vi "My Custom Controls - Custom.vi"() -> ()   [LabVIEW 2016]
doc: "Sample numeric display item."
uses:
  <vilib>/NI Veristand/Display Template Support/Display Template Support.llb/cluster_Screen Item Settings.ctl
  <vilib>/NI Veristand/Display Template Support/Display Template Support.llb/cluster_Graph Scale Settings.ctl
  <vilib>/NI Veristand/Display Template Support/Display Template Support.llb/cluster_Graph Plot Settings.ctl
  _typedefs/Custom Control_Data.ctl
  <vilib>/NI Veristand/Display Template Support/Display Template Support.llb/enum_Display Template Handler Minimal To Widget Msg.ctl
  <vilib>/NI Veristand/Display Template Support/Display Template Support.llb/enum_Display Template Handler Minimal To Workspace.ctl
  <vilib>/NI Veristand/Display Template Support/Display Template Support.llb/sub_Display Template Handler Custom.vi
panel:
  out "Custom Control - Data":T1
  in  "timeout":i32=-1
  in  "Custom Data":T1
  in  "Item.Data":T2
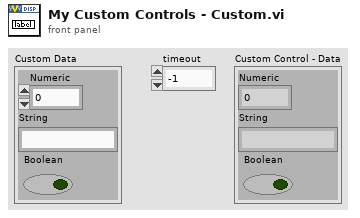
[diagram p1: front panel]
types:
  T1 = typedef "Custom Control_Data.ctl" = cluster{"Numeric":dbl, "String":string, "Boolean":bool}
  T2 = typedef "cluster_Screen Item Settings.ctl" = cluster{"Template VI":string, "Position X":i32, "Position Y":i32, "Custom":string, "Show Title Bar":bool, "ID":i32, "Always On Top":bool, "Allow Resize":bool, "Allow Minimize":bool, "Allow Close":bool, "Size to Screen":bool, "Screen.ID":i32, "State":enum16{"Normal", "New"}, "Title":string, "Window Bounds":cluster{"[0]":i16, "[1]":i16, "[2]":i16, "[3]":i16}, "Channel Ref":u64, "Unit":string, "Default Units?":bool, "Flash Limit?":bool, "Color 1":u32, "Color 2":u32, "Color 3":u32, "Color 4":u32, "Bck Color":u32, "Fore Color":u32, "Limit 1":dbl, "Limit 2":dbl, "Limit 3":dbl, "Limit 4":dbl, "Limit Mode 1":i32, "Limit Mode 2":i32, "Limit Mode 3":i32, "Limit Mode 4":i32, "Scale Precision":i32, "Scale Min":dbl, "Scale Max":dbl, "Format":i32, "Precision":i32, "Background Type":i32, "IDs":i32[], "Units":string[], "Labels":string[], "Scale Factor":dbl, "Scale Offset":dbl, "YScale Index":u32[], "XScale":T3, "YScales":T3[], "Plots":T4[], "Update Period":dbl, "History Length":dbl, "My.Ref":refnum<vi>, "Is Control?":bool, "Channel Paths":string[], "Custom Data":variant}
  T3 = typedef "cluster_Graph Scale Settings.ctl" = cluster{"Format":u8, "Precision":u8, "Fit":u8, "Label":string, "Use Default Label":bool, "Label Visible":bool, "Min":dbl, "Max":dbl}
  T4 = typedef "cluster_Graph Plot Settings.ctl" = cluster{"Bar Style":u8, "Fill To":i16, "Fill/PtColor":u32, "Line Style":u8, "Line Width":u8, "Color":u32, "Interp":u8, "Point Style":u8}
  T5 = typedef "enum_Display Template Handler Minimal To Workspace.ctl" = cluster{"Operation":enum16{"SetCustomData", "DeleteItem"}, "Data":variant}
  T6 = typedef "enum_Display Template Handler Minimal To Widget Msg.ctl" = enum16{"Stop", "LaunchConfigDialog"}
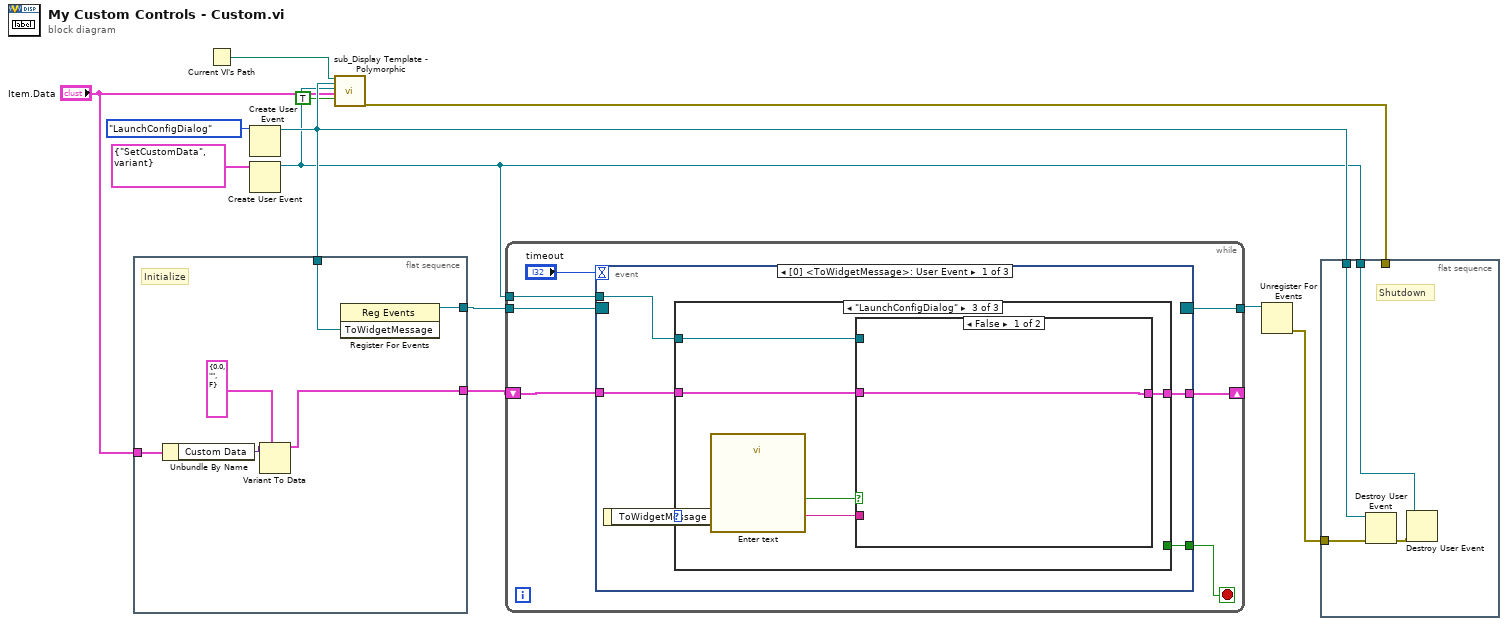
[diagram p0: block diagram]
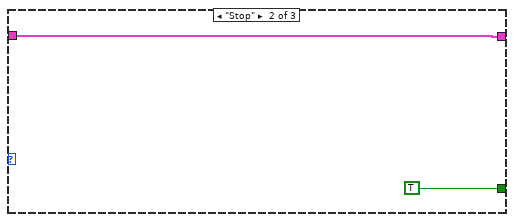
[diagram p3: hidden frame]
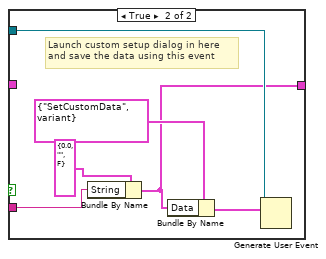
[diagram p4: hidden frame]
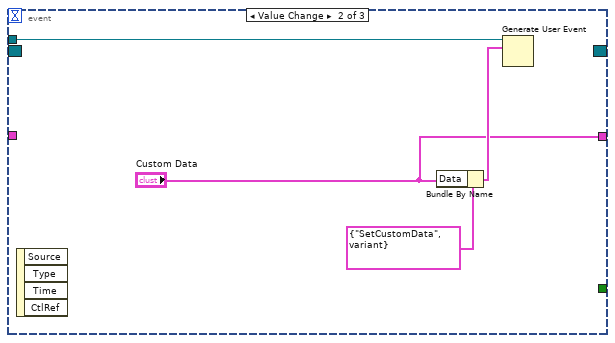
[diagram p5: hidden frame]
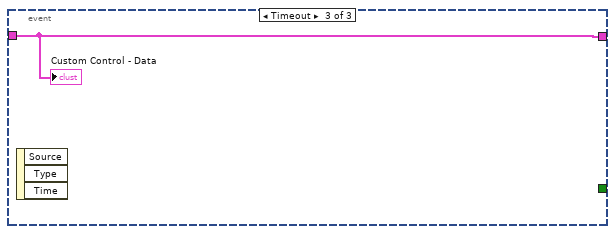
[diagram p6: hidden frame]
diagram:
  n1 = flat-sequence {
    tunnel: [w18] -> w10
    tunnel: w7 -> [w17]
    tunnel: "Item.Data" -> [w16]
    tunnel: [w13] -> w1
    frame #0 {
      # "Initialize"
      n2 = Unbundle By Name(w16) -> ("Custom Data"=w15:variant)
      n3 = Variant To Data(type=T1 {"Numeric"=0.0, "String"="", "Boolean"=FALSE}, Variant=w15) -> (data=w13:T1)  [unwired: 1 in, 1 out]
      n4 = register-events(w17) -> (reference out=w18:refnum<event-registration>)  [unwired: 2 in, 1 out]
    }
  }
  n5 = Current VI's Path() -> (path=w5:path)
  n6 = Create User Event(user event datatype=enum_Display_Template_Handler_Minimal_To_Widget_Msg."LaunchConfigDialog" ("ToWidgetMessage")) -> (user event=w7:refnum<user-event>)  [unwired: 1 in, 1 out]
  n7 = Create User Event(user event datatype=T5 {"Operation"=enum."SetCustomData", "Data"=variant} ("Data")) -> (user event=w3:refnum<user-event>)  [unwired: 1 in, 1 out]
  n8 = call-poly <vilib>:"sub_Display Template - Polymorphic.vi"("Parent.Path"=w5, "ToWidgetEvent"=w7, "ToWorkspace"=w3, "Item.Data"="Item.Data", "Resizable"=TRUE) -> ("error out"=w12:errorcluster)  [unwired: 1 in, 13 out]
  n9 = while {
    tunnel: w10 -> [w25]
    tunnel: [w23] -> w9
    tunnel: w3 -> [w22]
    shift-right: [w20] -> _
    shift-left: w1 -> [w21]
    stop <- w24 stop-if-true
    n10 = event shown="[0] <ToWidgetMessage>: User Event" {
      selector: w25 -> [_ _ _]
      dyn-events: [_ _ _] -> w23
      timeout: "timeout" -> [_ _ _]
      tunnel: [w29 _ _] -> w24
      tunnel: w22 -> [w28 w49 _]
      tunnel: w21 -> [w27 _ w50]
      tunnel: [w26 "Custom Data" w50] -> w20
      event User Event {
        n11 = event-data() -> ("ToWidgetMessage"=w30:T6)  [unwired: 1 out]
        n12 = case shown="\"LaunchConfigDialog\"" w30 {
          tunnel: [_ TRUE _] -> w29
          tunnel: w28 -> [_ _ w38]
          tunnel: w27 -> [w31 w32 w35]
          tunnel: [w31 w32 w34] -> w26
          frame Default {
          }
          frame "Stop" {
          }
          frame "LaunchConfigDialog" {
            n13 = call "Enter text"() -> ("Text"=w36:string, "OK"=w37:bool)  [unwired: 17 in, 1 out]
            n14 = case shown="False" w37 {
              tunnel: w38 -> [_ w45]
              tunnel: w36 -> [_ w41]
              tunnel: w35 -> [w39 _]
              tunnel: [w39 w40] -> w34
              frame False {
              }
              frame True {
                # "Launch custom setup dialog in here\nand save the data using this event"
                n15 = Bundle By Name(cluster=T1 {"Numeric"=0.0, "String"="", "Boolean"=FALSE}, "String"=w41) -> (w40:T1)
                n16 = Bundle By Name(cluster=T5 {"Operation"=enum."SetCustomData", "Data"=variant} ("event data"), "Data"=w40) -> (w43:T5)
                n17 = Generate User Event(user event=w45, event data cluster=w43) -> ()  [unwired: 2 in, 2 out]
              }
            }
          }
        }
      }
      event Value Change {
        n18 = event-data() -> ()  [unwired: 5 out]
        n19 = Bundle By Name(cluster=T5 {"Operation"=enum."SetCustomData", "Data"=variant} ("event data"), "Data"="Custom Data") -> (w47:T5)
        n20 = Generate User Event(user event=w49, event data cluster=w47) -> ()  [unwired: 2 in, 2 out]
      }
      event Timeout {
        n21 = event-data() -> ()  [unwired: 4 out]
        "Custom Control - Data" <- w50
      }
    }
  }
  n22 = Unregister For Events(event registration refnum=w9) -> (error out=w8:errorcluster)  [unwired: 1 in]
  n23 = flat-sequence {
    tunnel: w12 -> [_]
    tunnel: w8 -> [w53]
    tunnel: w7 -> [w54]
    tunnel: w3 -> [w51]
    frame #0 {
      # "Shutdown"
      n24 = Destroy User Event(user event=w54, error in=w53) -> (error out=w52:errorcluster)
      n25 = Destroy User Event(user event=w51, error in=w52) -> ()  [unwired: 1 out]
    }
  }
